vi "Global Settings.vi"() -> ()   [LabVIEW 2025]
panel:
  in  "Draw Menu Drag Indicator":refnum<vi>[](array[refnum])
  in  "Icon Scale Factor":dbl=0.75
  in  "Stoopid Fast Min %":dbl=90.0
  in  "Draw Arrows":bool=TRUE
  in  "Turn Angle Limit (deg)":dbl=90.0
  in  "> 90?":bool=TRUE
  in  "Field Size":cluster{"width":dbl, "height":dbl}={"width"=26.9166666667, "height"=35.2141666667}
  in  "Arrow Color":u32(colorbox)=14421504
  in  "Robot Rect":cluster{"x":dbl, "y":dbl, "x":dbl, "y":dbl}={"x"=-1.5208, "y"=-1.4375, "x"=1.5208, "y"=1.4375}
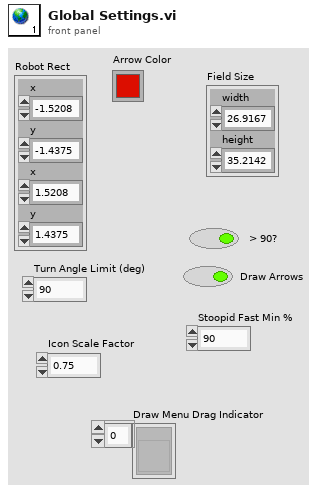
[diagram p1: front panel]
diagram:
